vi "Create Work Channel Endpoint.vi"(3 "Bundler Terminal":refnum<vi>, 4 "Channel Index":i32, 5 "Status CAR":refnum<vi>, 6 "Lossy":bool, 7 "Input CAR":refnum<vi>, 8 "Terminal Config":T1, 9 "Terminal":refnum<vi>, 10 "Frames[]":refnum<vi>[](array[refnum]), 11 "Index":i32) -> (0 "error out":errorcluster)   [LabVIEW 2020, in "FlexBlocks.lvlib"]
uses:
  FlexBlocks.lvlib
  Terminal Config.ctl
  Type Descriptor.ctl
  Terminal Direction.ctl
  Value Mode.ctl
  Special Terminal.ctl
  Terminal Mode.ctl
  <vilib>/Utility/miscctls.llb/LVPointTypeDef.ctl
  Lossy Terminal Index.ctl
  Lossless Terminal Index.ctl
  Status Terminal Index.ctl
panel:
  out "Value Terminal":refnum<vi>
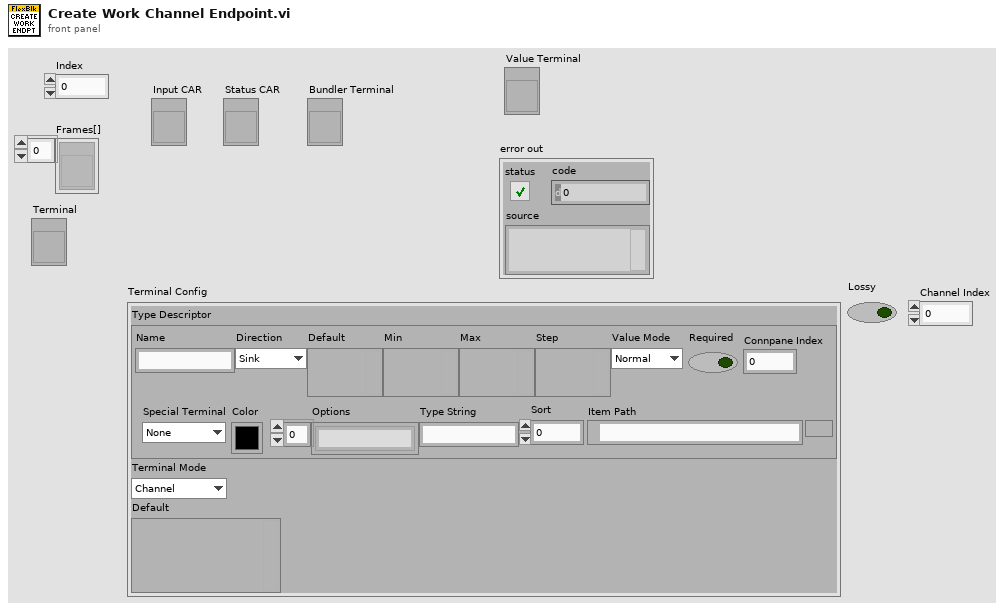
[diagram p1: front panel]
types:
  T1 = typedef "FlexBlocks.lvlib/Terminal Config.ctl" = cluster{"Type Descriptor":T2, "Terminal Mode":T6, "Default":variant}
  T2 = typedef "FlexBlocks.lvlib/Type Descriptor.ctl" = cluster{"Name":string, "Direction":T3, "Default":variant, "Min":variant, "Max":variant, "Step":variant, "Value Mode":T4, "Required":bool, "Connpane Index":i32, "Special Terminal":T5, "Color":u32, "Options":string[], "Type String":string, "Sort":i32, "Item Path":path}
  T3 = typedef "FlexBlocks.lvlib/Terminal Direction.ctl" = enum16{"Sink", "Source"}
  T4 = typedef "FlexBlocks.lvlib/Value Mode.ctl" = enum16{"Normal", "Range", "Select"}
  T5 = typedef "FlexBlocks.lvlib/Special Terminal.ctl" = enum16{"None", "Action", "Init", "Tag", "State in", "State out", "Error"}
  T6 = typedef "FlexBlocks.lvlib/Terminal Mode.ctl" = enum16{"Channel", "Config", "Value", "Control Ref"}
  T7 = typedef "FlexBlocks.lvlib/Status Terminal Index.ctl" = enum16{"# Pending Write", "# Pending Read", "Usage Ratio (0-1)", "# Queued", "Closed", "Updated Time", "N/A 6", "Sequence #", "N/A 8", "N/A 9", "N/A 10", "FlexChannel"}
  T8 = typedef "FlexBlocks.lvlib/Lossless Terminal Index.ctl" = enum16{"Depth", "Timeout mS", "FlexChannel", "Release", "N/A 4", "Timed Out", "N/A 6", "Value", "Closed", "N/A 9"}
  T9 = typedef "FlexBlocks.lvlib/Lossy Terminal Index.ctl" = enum16{"Wait for Next", "Updated Time", "FlexChannel", "Wait Timeout mS", "Sequence #", "Timed Out", "N/A 6", "Value", "Closed", "N/A 9"}
  T10 = typedef "LVPointTypeDef.ctl" = cluster{"Horizontal":i16, "Vertical":i16}
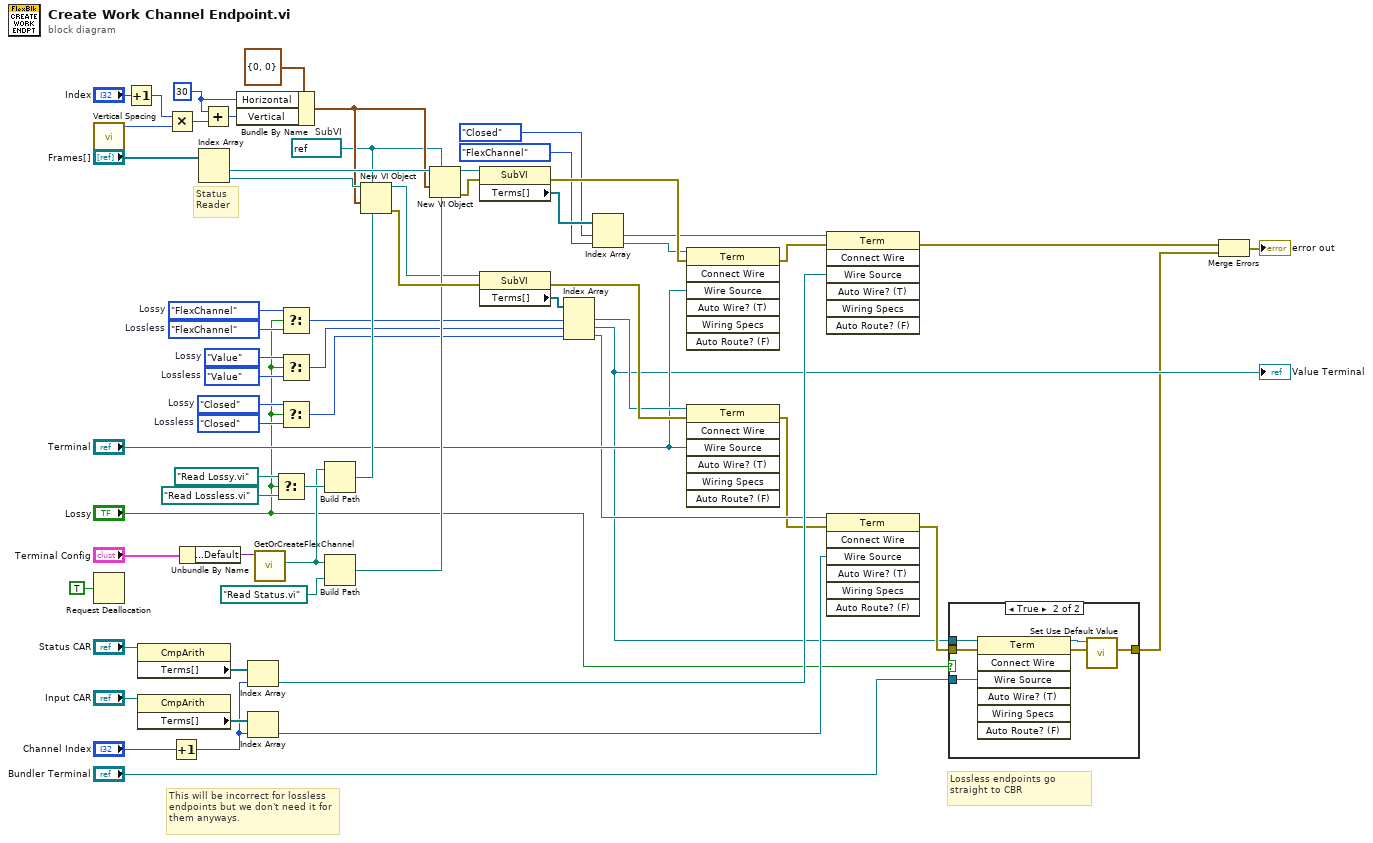
[diagram p0: block diagram]
diagram:
  w35 = Lossless_Terminal_Index."Closed"  # Lossless
  w34 = Lossy_Terminal_Index."Closed"  # Lossy
  w37 = Lossless_Terminal_Index."Value"  # Lossless
  w36 = Lossy_Terminal_Index."Value"  # Lossy
  w38 = Lossless_Terminal_Index."FlexChannel"  # Lossless
  w39 = Lossy_Terminal_Index."FlexChannel"  # Lossy
  w6 = 30 ("Left")
  w42 = refnum<vi> refnum  # SubVI
  # "This will be incorrect for lossless endpoints but we don't need it for them anyways."
  # "Lossless endpoints go straight to CBR"
  # "Status\nReader"
  n1 = call "Vertical Spacing.vi"() -> ("Spacing"=w45:i32)  [unwired: 11 in]
  n2 = Request Deallocation(TRUE ("flag")) -> ()
  n3 = Increment(x="Index") -> (x+1=w52:i32)
  n4 = property class="CmpArith"(reference="Status CAR") -> ("Terms[]"=w20:refnum<vi>[])  [unwired: 1 in, 2 out]
  n5 = property class="CmpArith"(reference="Input CAR") -> ("Terms[]"=w19:refnum<vi>[])  [unwired: 1 in, 2 out]
  n6 = Multiply(x=w52, y=w45) -> (x*y=w8:i32)
  n7 = Increment(x="Channel Index") -> (x+1=w17:i32)
  n8 = Unbundle By Name("Terminal Config") -> ("Type Descriptor.Default"=w56:variant)
  n9 = Index Array(array="Frames[]") -> (element #1=w58:refnum<vi>, element #2=w47:refnum<vi>)  [unwired: 2 in]
  n10 = Add(x=w6, y=w8) -> (x+y=w7:i32)
  n11 = Bundle By Name(cluster=T10 {"Horizontal"=0, "Vertical"=0} ("location"), "Horizontal"=w6, "Vertical"=w7) -> (w43:T10)
  n12 = Index Array(array=w20, index=w17) -> (element=w15:refnum<vi>)
  n13 = Index Array(array=w19, index=w17) -> (element=w12:refnum<vi>)
  n14 = call "GetOrCreateFlexChannel.vi"("Element Type"=w56) -> ("Channel Folder"=w48:path)  [unwired: 8 in, 2 out]
  n15 = Select(t=path "Read Lossy.vi" ("name or relative path"), s="Lossy", f=path "Read Lossless.vi" ("name or relative path")) -> (s? t:f=w49:path)
  n16 = Select(t=w39, s="Lossy", f=w38) -> (s? t:f=w33:u16)
  n17 = Select(t=w36, s="Lossy", f=w37) -> (s? t:f=w32:u16)
  n18 = Select(t=w34, s="Lossy", f=w35) -> (s? t:f=w31:u16)
  n19 = Build Path(base path=w48, name or relative path=w49) -> (appended path=w46:path)
  n20 = Build Path(base path=w48, name or relative path=path "Read Status.vi") -> (appended path=w54:path)
  n21 = New VI Object(vi object class=w42, owner refnum=w47, position/next to=w43, 6:w46) -> (object refnum=w41:refnum<vi>, 0:w62:errorcluster)  [unwired: 4 in]
  n22 = New VI Object(vi object class=w42, owner refnum=w58, position/next to=w43, 6:w54) -> (object refnum=w29:refnum<vi>, 0:w28:errorcluster)  [unwired: 4 in]
  n23 = property class="SubVI"(reference=w29, error in=w28) -> (error out=w63:errorcluster, "Terms[]"=w27:refnum<vi>[])  [unwired: 1 out]
  n24 = property class="SubVI"(reference=w41, error in=w62) -> (error out=w61:errorcluster, "Terms[]"=w40:refnum<vi>[])  [unwired: 1 out]
  n25 = Index Array(array=w40, index #1=w33, index #2=w32, index #3=w31) -> (element #1=w30:refnum<vi>, element #2=w4:refnum<vi>, element #3=w13:refnum<vi>)
  "Value Terminal" <- w4
  n26 = Index Array(array=w27, index #1=Status_Terminal_Index."Closed" ("Status Terminal Index"), index #2=Status_Terminal_Index."FlexChannel" ("Status Terminal Index")) -> (element #1=w16:refnum<vi>, element #2=w23:refnum<vi>)
  n27 = invoke class="Term" method="Connect Wire"(reference=w23, error in=w63, "Wire Source"="Terminal") -> (error out=w14:errorcluster)  [unwired: 4 in, 6 out]
  n28 = invoke class="Term" method="Connect Wire"(reference=w30, error in=w61, "Wire Source"="Terminal") -> (error out=w11:errorcluster)  [unwired: 4 in, 6 out]
  n29 = invoke class="Term" method="Connect Wire"(reference=w16, error in=w14, "Wire Source"=w15) -> (error out=w10:errorcluster)  [unwired: 4 in, 6 out]
  n30 = invoke class="Term" method="Connect Wire"(reference=w13, error in=w11, "Wire Source"=w12) -> (error out=w5:errorcluster)  [unwired: 4 in, 6 out]
  n31 = case shown="True" "Lossy" {
    tunnel: w5 -> [w64 w70]
    tunnel: w4 -> [_ w69]
    tunnel: "Bundler Terminal" -> [_ w68]
    tunnel: [w64 w65] -> w1
    frame False {
    }
    frame True {
      n32 = invoke class="Term" method="Connect Wire"(reference=w69, error in=w70, "Wire Source"=w68) -> (reference out=w66:refnum<vi>, error out=w67:errorcluster)  [unwired: 4 in, 5 out]
      n33 = call "Set Use Default Value.vi"("error in (no error)"=w67, "Terminal"=w66) -> ("error out"=w65:errorcluster)  [unwired: 9 in]
    }
  }
  n34 = Merge Errors(w10, w1) -> (→"error out":errorcluster)
